vi "WorspacePathGenerator.vi"() -> (3 "appended path":path)   [LabVIEW 2017]
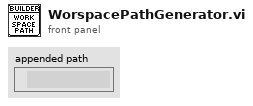
[diagram p1: front panel]
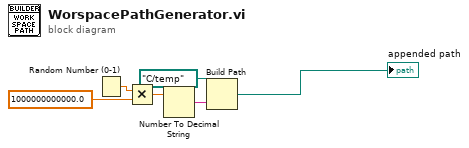
[diagram p0: block diagram]
diagram:
  n1 = Random Number (0-1)() -> (number: 0 to 1=w1:dbl)
  n2 = Multiply(x=w1, y=1000000000000.0) -> (x*y=w3:dbl)
  n3 = Number To Decimal String(number=w3) -> (decimal integer string=w4:string)  [unwired: 1 in]
  n4 = Build Path(base path=path "C:/temp", name or relative path=w4) -> (appended path=→"appended path":path)
